vi "Layout FGV.vi"(7 "String":string, 8 "Variant":variant, 9 "name":string, 10 "file (use dialog)":path, 11 "InitRef":T1) -> ()   [LabVIEW 2020, in "MDI ViewManager.lvlib"]
uses:
  MDI ViewManager.lvlib
  <vilib>/Utility/miscctls.llb/LVPointTypeDef.ctl
  <vilib>/Utility/miscctls.llb/LVBoundsTypeDef.ctl
  <vilib>/Utility/miscctls.llb/LVPositionTypeDef.ctl
  Typedef/Update ViewList.ctl
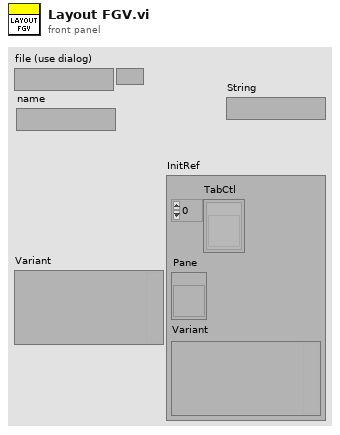
[diagram p1: front panel]
types:
  T1 = cluster{"TabCtl":refnum<vi>[], "Pane":refnum<vi>, "Variant":variant}
  T2 = typedef "LVPointTypeDef.ctl" = cluster{"Horizontal":i16, "Vertical":i16}
  T3 = typedef "LVBoundsTypeDef.ctl" = cluster{"Width":u32, "Height":u32}
  T4 = typedef "LVPositionTypeDef.ctl" = cluster{"Left":i32, "Top":i32}
  T5 = cluster{"Origin":T2, "Layout":cluster{"Pane Dimension":T3, "Position":T4, "Label":string, "Visible":bool, "InsertedViewName":string}[]}
  T6 = typedef "MDI ViewManager.lvlib/Update ViewList.ctl" = cluster{"Name":string, "VIPath":path, "Height(Default)":u32, "Widht(Default)":u32, "VIRef":refnum<vi>}
  T7 = cluster{"Pane Dimension":T3, "Position":T4, "Label":string, "Visible":bool, "InsertedViewName":string}
  T8 = cluster{"Pane Dimension":T3, "Position":T4, "Label":string, "Visible":bool, "InsertedViewName":string}[]
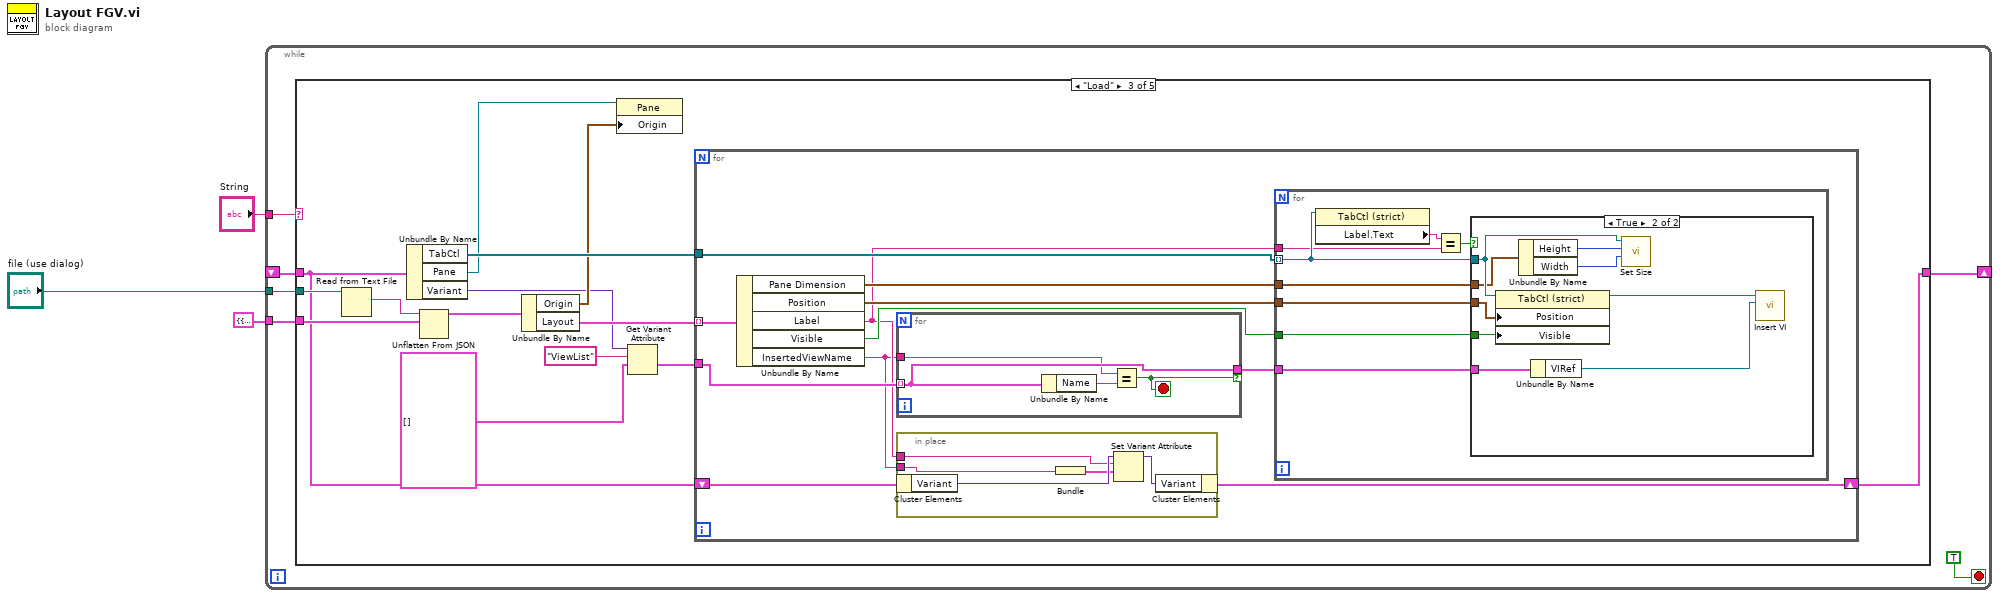
[diagram p0: block diagram]
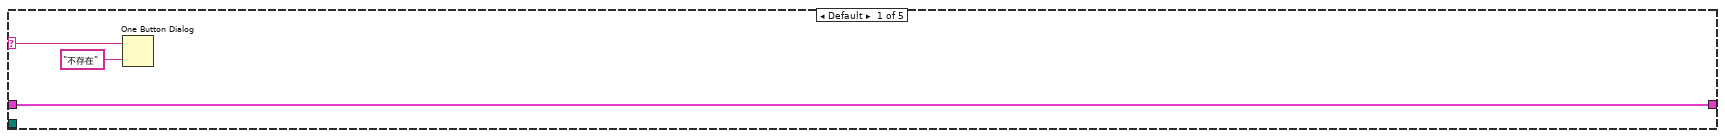
[diagram p2: hidden frame]
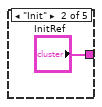
[diagram p3: hidden frame]
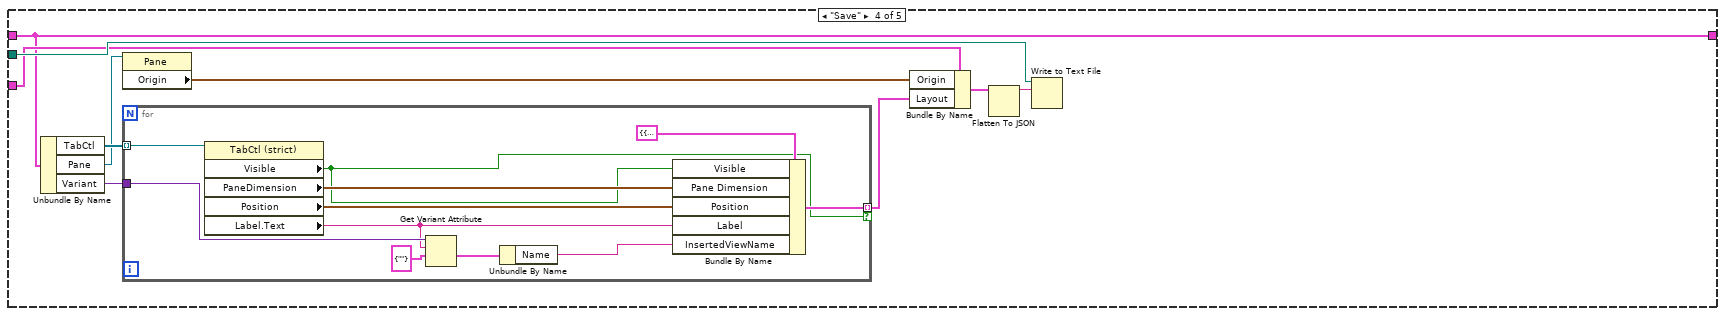
[diagram p5: hidden frame]
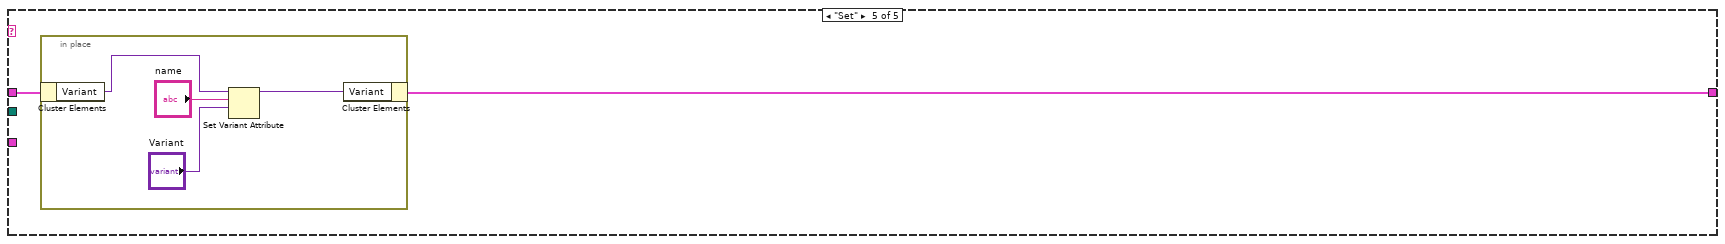
[diagram p6: hidden frame]
diagram:
  n1 = while {
    tunnel: "String" -> [w7]
    tunnel: "file (use dialog)" -> [w6]
    shift-right: [w5] -> _
    shift-left: _ -> [w8]
    tunnel: T5 {"Origin"={"Horizontal"=0, "Vertical"=0}, "Layout"=[]} -> [w4]
    stop <- TRUE stop-if-true
    n2 = case shown="\"Load\"" w7 {
      selector: w7 -> [w11 _ _ _ _]
      tunnel: w8 -> [w12 _ w16 w68 w87]
      tunnel: w6 -> [_ _ w26 w73 _]
      tunnel: [w12 "InitRef" w15 w68 w86] -> w5
      tunnel: w4 -> [_ _ w25 w69 _]
      frame Default {
        n3 = One Button Dialog(message=w11, button name ("OK")="不存在") -> ()  [unwired: 1 out]
      }
      frame "Init" {
      }
      frame "Load" {
        n4 = Read from Text File(file (use dialog)=w26) -> (text=w27:string)  [unwired: 3 in, 3 out]
        n5 = Unbundle By Name(w16) -> ("TabCtl"=w22:refnum<vi>[], "Pane"=w21:refnum<vi>, "Variant"=w19:variant)
        n6 = Unflatten From JSON(JSON string=w27, type and defaults=w25) -> (value=w24:T5)  [unwired: 5 in, 1 out]
        n7 = Unbundle By Name(w24) -> ("Origin"=w20:T2, "Layout"=w23:T8)
        n8 = property class="Pane"(reference=w21, "Origin"=w20) -> ()  [unwired: 1 in, 2 out]
        n9 = Get Variant Attribute(Variant=w19, name="ViewList", default value (empty Variant)=T6[] [] ("1.Val.UpdateInsertableVI")) -> (value=w14:T6[])  [unwired: 1 in, 3 out]
        n10 = for {
          tunnel: w23 -> [w37] mode=indexing
          tunnel: w22 -> [w38]
          tunnel: w14 -> [w33]
          shift-right: [w30] -> w15
          shift-left: w16 -> [w31]
          n11 = Unbundle By Name(w37) -> ("Pane Dimension"=w36:T3, "Position"=w35:T4, "Label"=w29:string, "Visible"=w34:bool, "InsertedViewName"=w28:string)
          n12 = for {
            tunnel: w33 -> [w47] mode=indexing
            tunnel: [w47] -> w32 if=w46
            tunnel: w28 -> [w45]
            stop <- w46 stop-if-true
            n13 = Unbundle By Name(w47) -> ("Name"=w44:string)
            n14 = Equal?(x=w45, y=w44) -> (x = y?=w46:bool)
          }
          n15 = in-place {
            in-place-border: w29 -> [w41]
            in-place-border: w28 -> [w40]
            n16 = in-place-cluster #1(w31) -> ("Variant"=w43:variant)
            n17 = Bundle("InsertedViewName"=w40) -> (w39:cluster{"InsertedViewName":string})  [unwired: 1 in]
            n18 = Set Variant Attribute(Variant=w43, name=w41, value=w39) -> (Variant out=w42:variant)  [unwired: 1 in, 2 out]
            n19 = in-place-cluster #1("Variant"=w42) -> (w30:T1)
          }
          n20 = for {
            tunnel: w38 -> [w55] mode=indexing
            tunnel: w36 -> [w52]
            tunnel: w35 -> [w51]
            tunnel: w29 -> [w50]
            tunnel: w34 -> [w49]
            tunnel: w32 -> [w48]
            n21 = property class="TabCtl (strict)"(reference=w55) -> ("Label.Text"=w54:string)  [unwired: 1 in, 2 out]
            n22 = Equal?(x=w54, y=w50) -> (x = y?=w53:bool)
            n23 = case shown="True" w53 {
              tunnel: w52 -> [_ w59]
              tunnel: w51 -> [_ w64]
              tunnel: w49 -> [_ w63]
              tunnel: w55 -> [_ w60]
              tunnel: w48 -> [_ w61]
              frame False {
              }
              frame True {
                n24 = property class="TabCtl (strict)"(reference=w60, "Position"=w64, "Visible"=w63) -> (reference out=w62:refnum<vi>)  [unwired: 1 in, 1 out]
                n25 = Unbundle By Name(w59) -> ("Height"=w58:u32, "Width"=w57:u32)
                n26 = Unbundle By Name(w61) -> ("VIRef"=w56:refnum<vi>)
                n27 = call "Set Size.vi"("Widht"=w57, "Height"=w58, "TabControlRef in"=w60) -> ()  [unwired: 7 in, 2 out]
                n28 = call "Insert VI.vi"("VIRef"=w56, "TabControl in"=w62) -> ()  [unwired: 8 in, 2 out]
              }
            }
          }
        }
      }
      frame "Save" {
        n29 = Unbundle By Name(w68) -> ("TabCtl"=w67:refnum<vi>[], "Pane"=w66:refnum<vi>, "Variant"=w65:variant)
        n30 = property class="Pane"(reference=w66) -> ("Origin"=w72:T2)  [unwired: 1 in, 2 out]
        n31 = for {
          tunnel: w67 -> [w80] mode=indexing
          tunnel: [w83] -> w71 mode=indexing if=w81
          tunnel: w65 -> [w79]
          n32 = property class="TabCtl (strict)"(reference=w80) -> ("Visible"=w81:bool, "PaneDimension"=w85:T3, "Position"=w84:T4, "Label.Text"=w78:string)  [unwired: 1 in, 2 out]
          n33 = Get Variant Attribute(Variant=w79, name=w78, default value (empty Variant)=cluster{"Name":string} {"Name"=""} ("output cluster")) -> (value=w76:cluster{"Name":string})  [unwired: 1 in, 3 out]
          n34 = Unbundle By Name(w76) -> ("Name"=w75:string)
          n35 = Bundle By Name(cluster=T7 {"Pane Dimension"={"Width"=0, "Height"=0}, "Position"={"Left"=0, "Top"=0}, "Label"="", "Visible"=FALSE, "InsertedViewName"=""}, "Visible"=w81, "Pane Dimension"=w85, "Position"=w84, "Label"=w78, "InsertedViewName"=w75) -> (w83:T7)
        }
        n36 = Bundle By Name(cluster=w69, "Origin"=w72, "Layout"=w71) -> (w70:T5)
        n37 = Flatten To JSON(anything=w70) -> (JSON string=w74:string)  [unwired: 2 in, 1 out]
        n38 = Write to Text File(file (use dialog)=w73, text=w74) -> ()  [unwired: 2 in, 3 out]
      }
      frame "Set" {
        n39 = in-place {
          n40 = in-place-cluster #2(w87) -> ("Variant"=w91:variant)
          n41 = Set Variant Attribute(Variant=w91, name="name", value="Variant") -> (Variant out=w90:variant)  [unwired: 1 in, 2 out]
          n42 = in-place-cluster #2("Variant"=w90) -> (w86:T1)
        }
      }
    }
  }
